vi "Set Macro String.vi"(8 "error in (no error)":errorcluster, 9 "Macro String":string, 10 "Macro Name":string, 11 "JKI SM in":refnum<class "JKI SM.lvclass">) -> (0 "error out":errorcluster, 3 "JKI SM out":refnum<class "JKI SM.lvclass">)   [LabVIEW 2013, in "JKI State Machine API.lvlib" / "JKI SM.lvclass"]
uses:
  JKI SM.lvclass
  JKI SM.lvclass/JKI SM.ctl
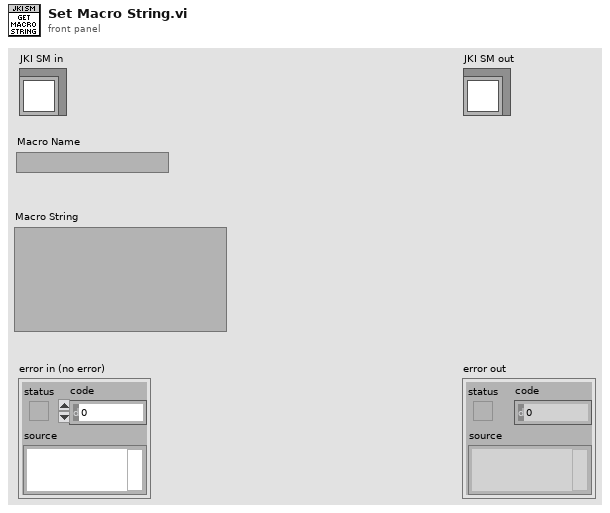
[diagram p1: front panel]
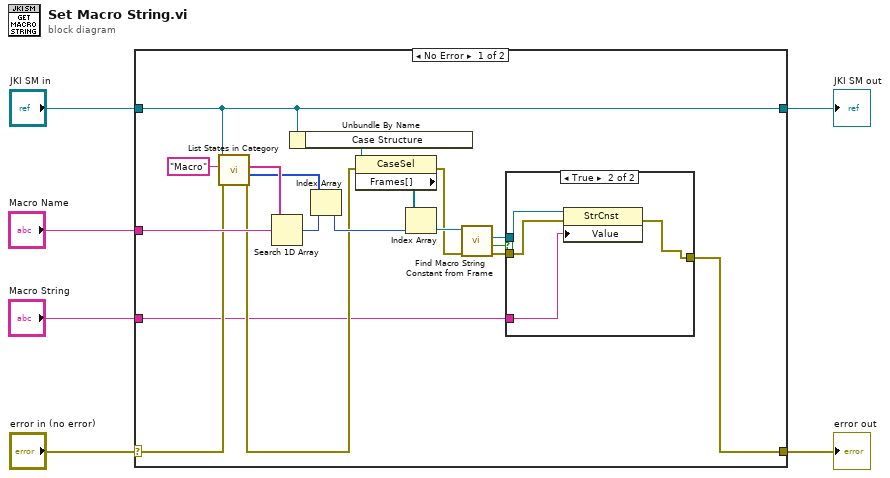
[diagram p0: block diagram]
diagram:
  n1 = case shown="No Error" "error in (no error)" {
    selector: "error in (no error)" -> [w19 w31]
    tunnel: [w9 w31] -> w5
    tunnel: [w18 w30] -> w3
    tunnel: "JKI SM in" -> [w18 w30]
    tunnel: "Macro Name" -> [w22 _]
    tunnel: "Macro String" -> [w7 _]
    frame No Error {
      n2 = call "List States in Category.vi"("error in (no error)"=w19, "Category"="Macro", "JKI SM in"=w18) -> ("error out"=w12:errorcluster, "State Frame Indices"=w21:i32[], "States"=w23:string[])  [unwired: 4 in, 2 out]
      n3 = Search 1D Array(1D array=w23, element=w22) -> (index of element=w20:i32)  [unwired: 1 in]
      n4 = Unbundle By Name(w18) -> ("Case Structure"=w17:refnum<vi>)
      n5 = Index Array(array=w21, index=w20) -> (element=w15:i32)
      n6 = property class="CaseSel"(reference=w17, error in=w12) -> (error out=w13:errorcluster, "Frames[]"=w16:refnum<vi>[])  [unwired: 1 out]
      n7 = Index Array(array=w16, index=w15) -> (element=w14:refnum<vi>)
      n8 = call "Find Macro String Constant from Frame.vi"("error in (no error)"=w13, "Diagram in"=w14) -> ("error out"=w10:errorcluster, "Found?"=w8:bool, "Macro String Constant"=w11:refnum<vi>)  [unwired: 6 in, 1 out]
      n9 = case shown="True" w8 {
        tunnel: w11 -> [_ w29]
        tunnel: w10 -> [w25 w28]
        tunnel: [w25 w27] -> w9
        tunnel: w7 -> [_ w26]
        frame False {
        }
        frame True {
          n10 = property class="StrCnst"(reference=w29, error in=w28, "Value"=w26) -> (error out=w27:errorcluster)  [unwired: 1 out]
        }
      }
    }
    frame Error {
    }
  }
  "error out" <- w5
  "JKI SM out" <- w3
